vi "kim - generate format string.vi"(7 "input string":string="%f", 10 "number":i32=9) -> (2 "format":string)   [LabVIEW 2015]
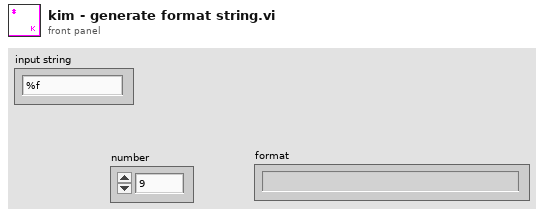
[diagram p1: front panel]
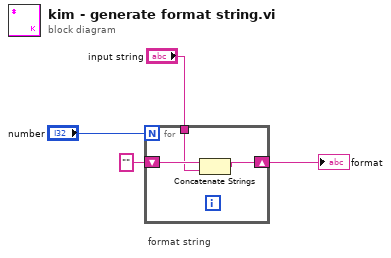
[diagram p0: block diagram]
diagram:
  # "format string"
  n1 = for {
    N: "number" -> [_]
    shift-right: [w7] -> w2
    shift-left: "" ("input string") -> [w6]
    tunnel: "input string" -> [w5]
    n2 = Concatenate Strings(w6, w5) -> (w7:string)
  }
  "format" <- w2
